vi "Process.vi"(8 "error in":errorcluster, 11 "Chart[Template]":refnum<class "Chart[Template].lvclass">) -> (0 "error out":errorcluster, 3 "Graph[Template] out":refnum<class "Chart[Template].lvclass">)   [LabVIEW 2013, in "Chart[Template].lvclass"]
doc: "---------------------------------------------------------------\nJKI State Machine Objects™\nhttp://jki.net/state-machine-objects/\nCopyright (C) 2005-2015, JKI <info@jki.net>\nALL RIGHTS RESERVEDJKI State Machine Objects (SMO) 1.0.0.5\nJKI - JKI\nCopyright (c) 2016, JKI"
uses:
  Chart[Template].lvclass
  <vilib>/JKI/JKI SMO/SMO/Typedefs/Parent Call--Enum.ctl
  <vilib>/JKI/JKI SMO/SMO.UI/SMO.UI.lvclass
  Chart[Template].lvclass/Chart[Template].ctl
  <vilib>/JKI/JKI SMO/SMO/SMO.lvclass
panel:
  in  "------------- Registered Events -------------":bool
  in  "------------- Public API -------------":bool
  out "Waveform Chart":dbl(graph)
  # "For instructions on how to use the JKI State Machine Objects, examples and video tutorials, visit:\nhttp://jki.net/state-machine-objects/\n\nJKI State Machine Objects™\nhttp://jki.net/state-machine-objects/\nCopyright (C) 2005-2015, JKI <info@jki.net>\nALL RIGHTS RESERVED"
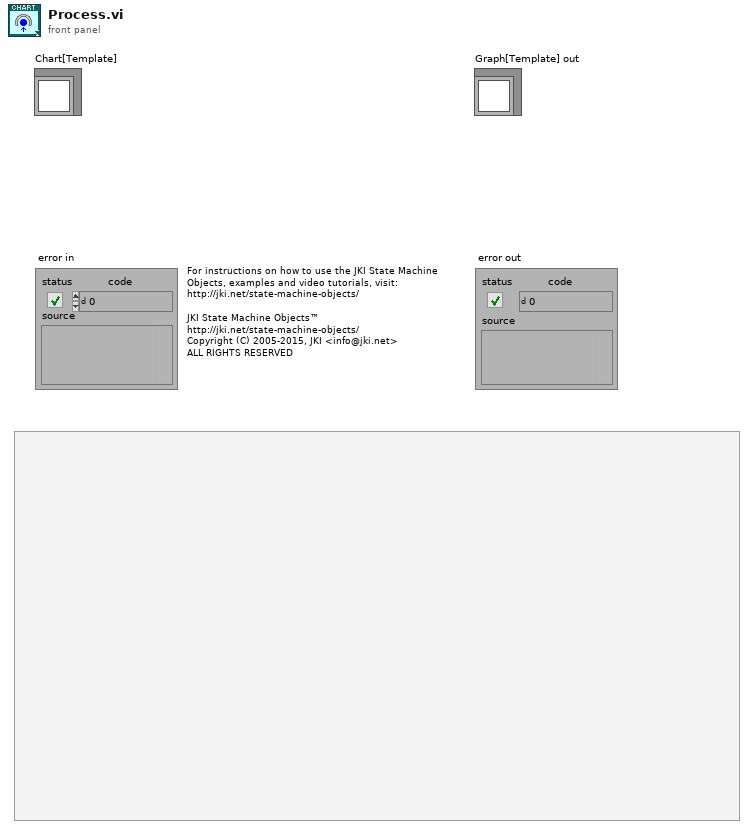
[diagram p1: front panel]
types:
  T1 = typedef "SMO.lvclass/Parent Call--Enum.ctl" = enum16{"Allows parent to run", "Does not request parent to run"}
  T2 = enum32{"invalid app kind", "Development System", "Run Time System", "Student Edition", "Embedded LabVIEW", "Evaluation", "Custom"}
  T3 = enum32{"Invalid", "Standard", "Closed", "Hidden", "Minimized", "Maximized"}
  T4 = cluster{"Core":cluster{"Current VI Reference":refnum<vi>, "Close Panel on Exit?":bool, "error":errorcluster}, "Self Reference":refnum<class "Chart[Template].lvclass">, "bool":bool}
  T5 = cluster{"Current VI Reference":refnum<vi>, "Close Panel on Exit?":bool, "error":errorcluster}
  T6 = typedef "SMO.lvclass/Protected Events.ctl" = cluster{"StopProcesses":refnum<user-event>, "AbortProcesses":refnum<user-event>, "Config Changed":refnum<user-event>}
  T7 = typedef "Chart[Template].lvclass/ProtectedEvents--Cluster.ctl" = cluster{"Clear Chart":refnum<user-event>}
  T8 = typedef "Chart[Template].lvclass/Dependencies--Cluster.ctl" = cluster{"SMO":refnum<class "SMO.lvclass">, "New Value":refnum<user-event>}
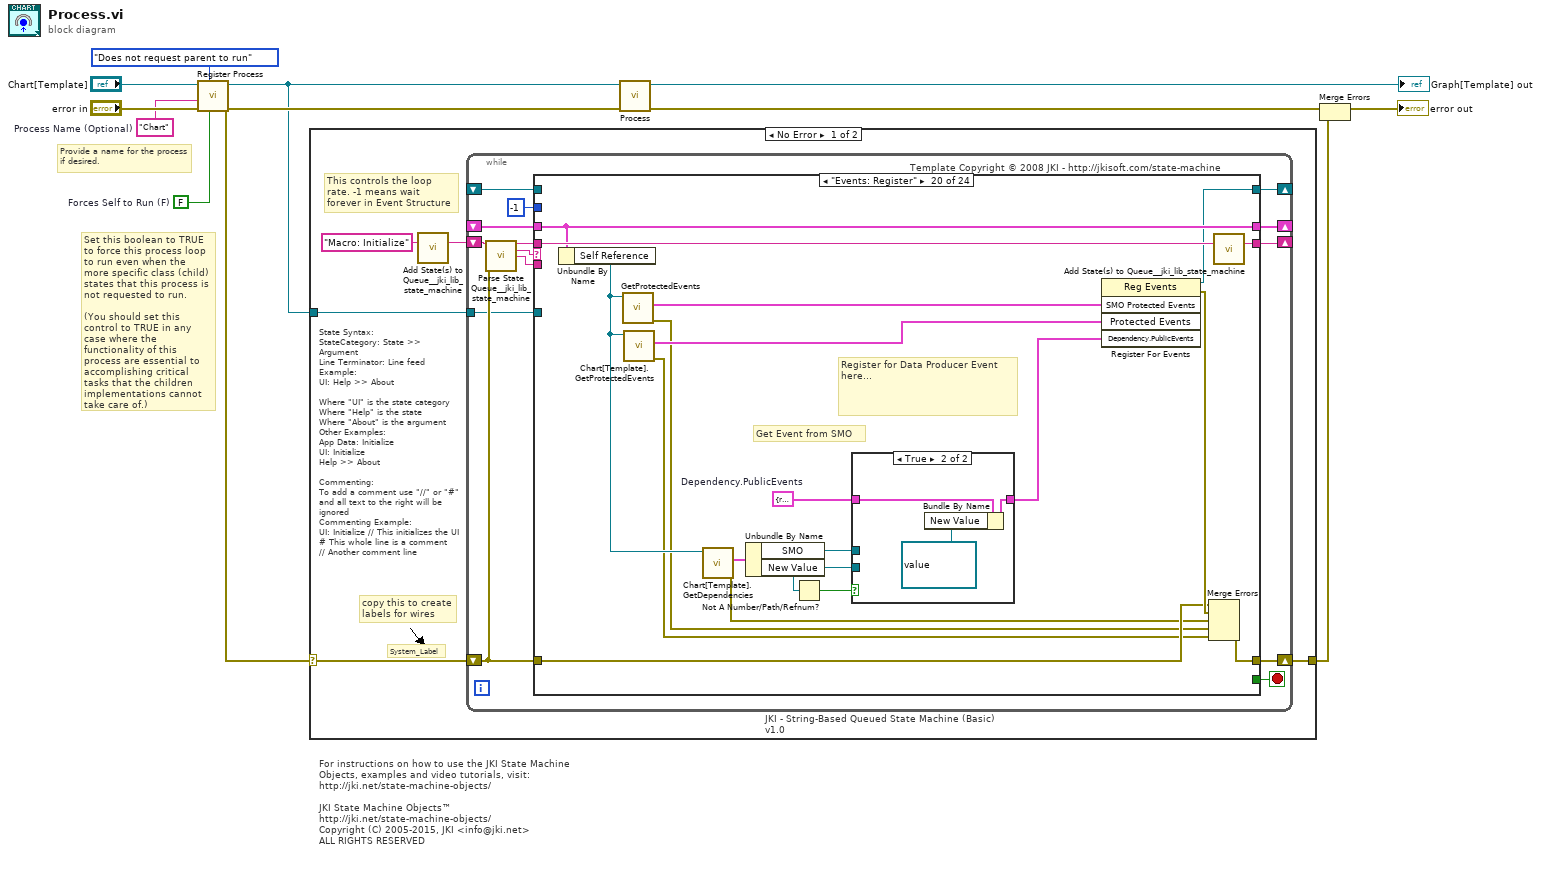
[diagram p0: block diagram]
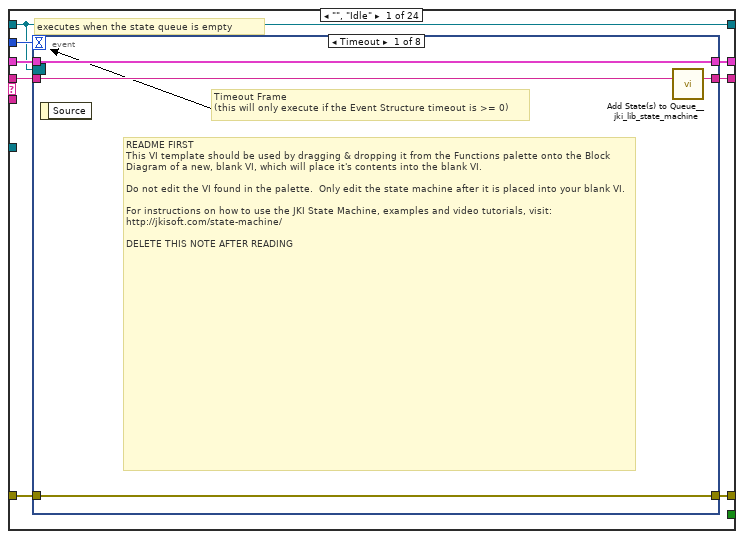
[diagram p2: hidden frame]
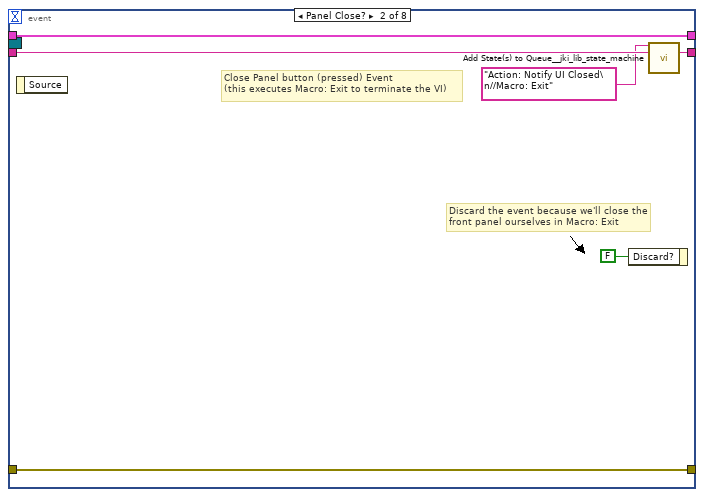
[diagram p3: hidden frame]
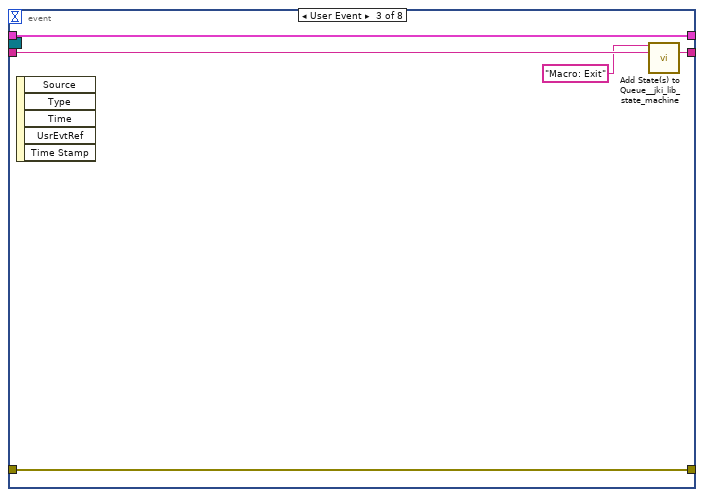
[diagram p4: hidden frame]
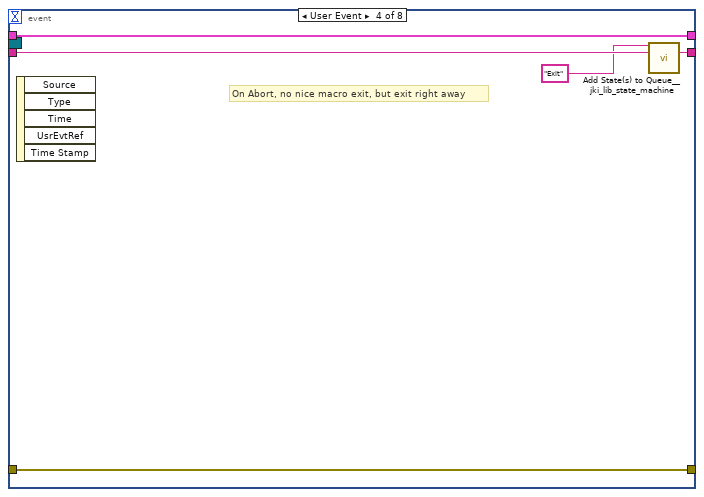
[diagram p5: hidden frame]
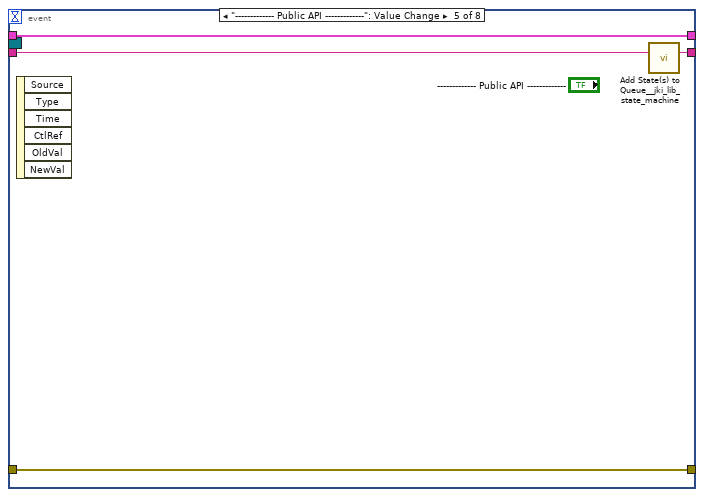
[diagram p6: hidden frame]
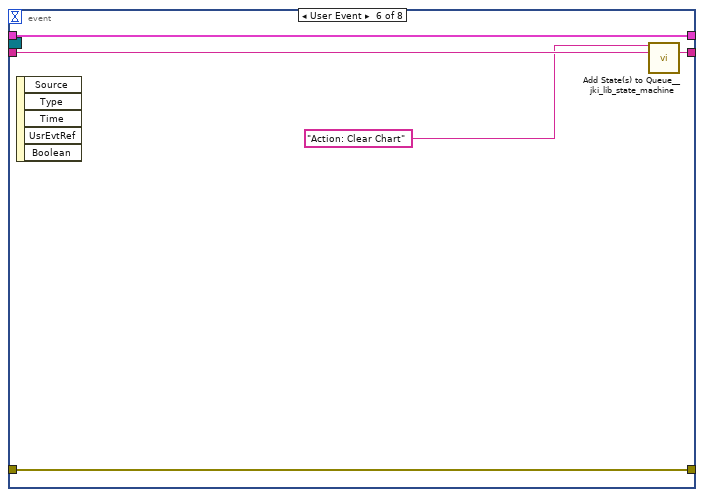
[diagram p7: hidden frame]
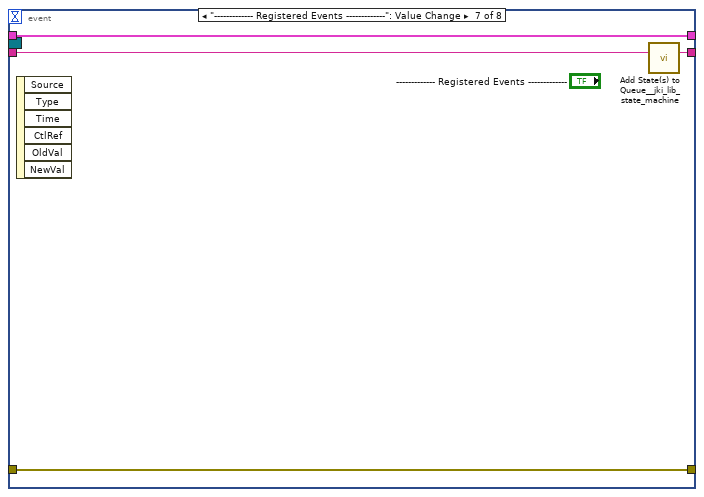
[diagram p8: hidden frame]
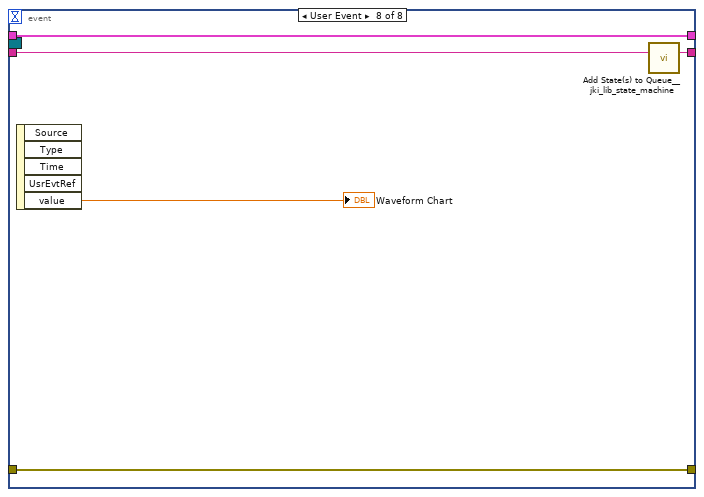
[diagram p9: hidden frame]
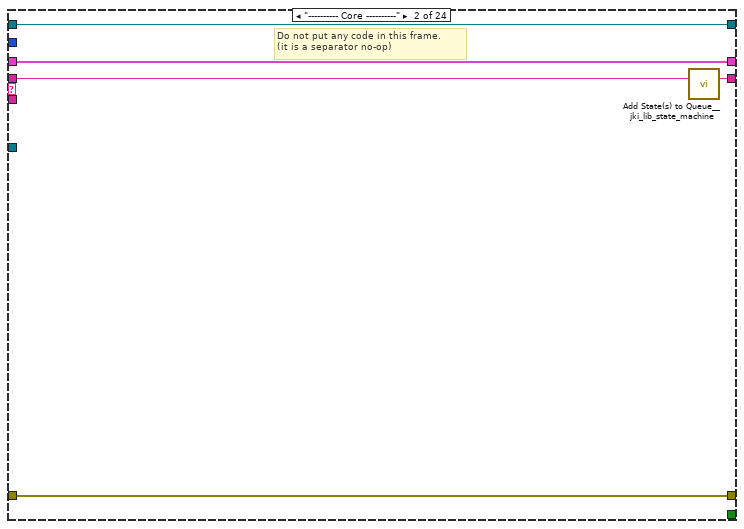
[diagram p10: hidden frame]
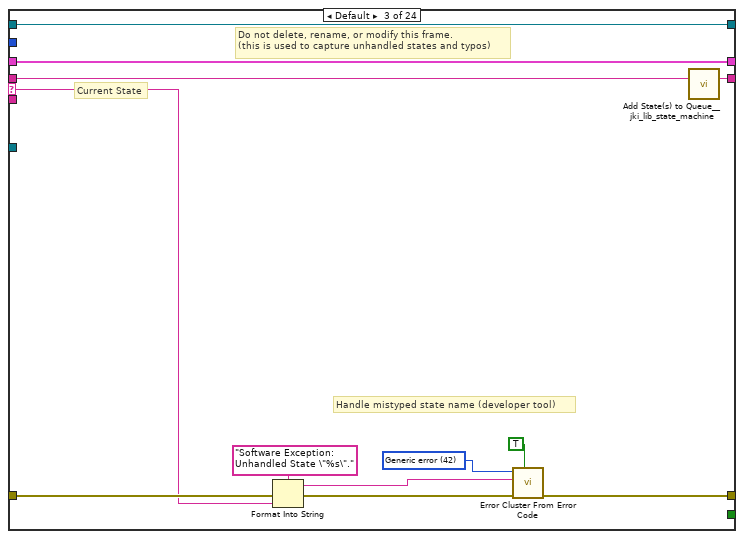
[diagram p11: hidden frame]
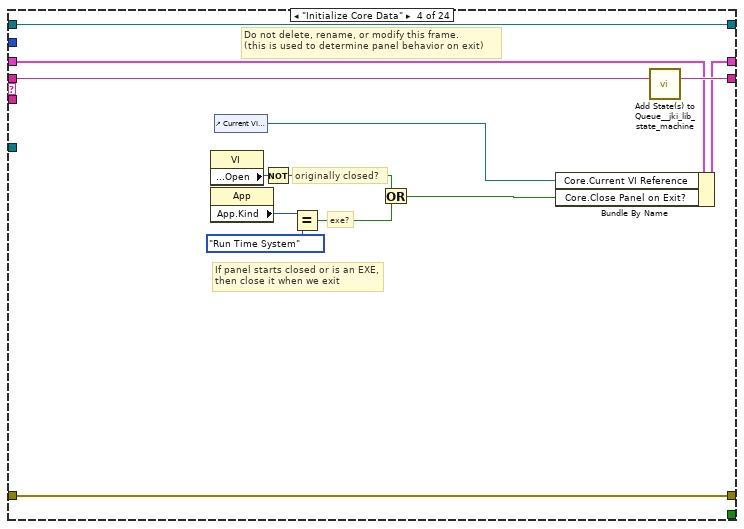
[diagram p12: hidden frame]
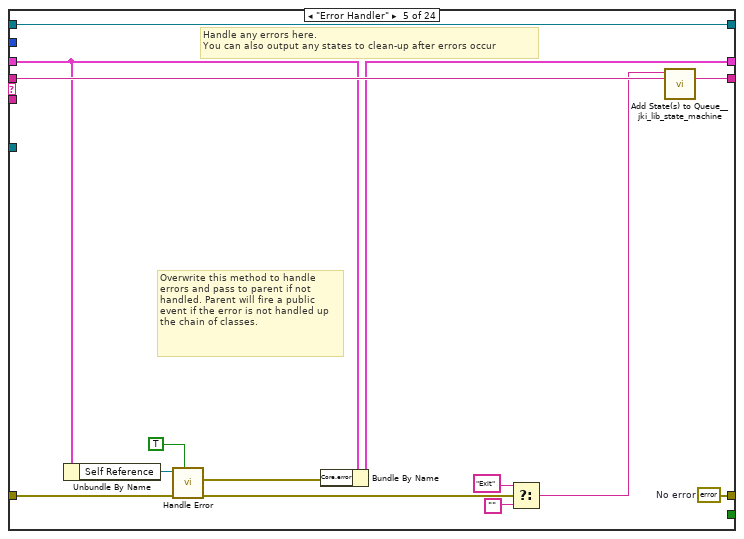
[diagram p13: hidden frame]
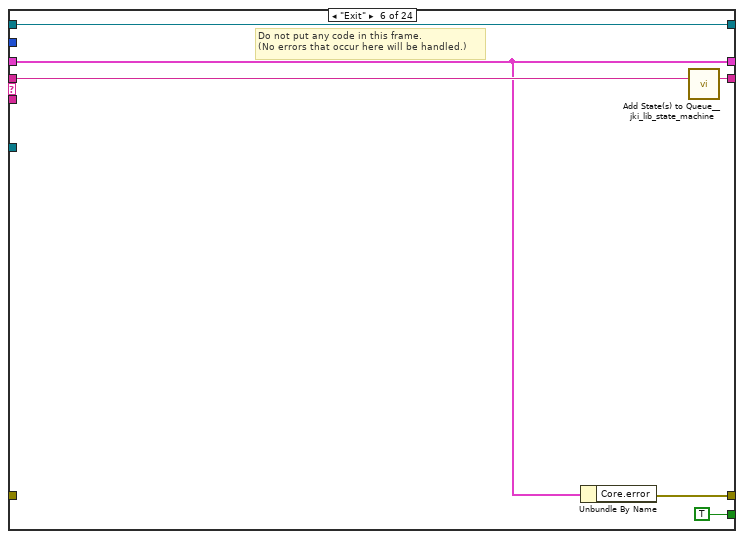
[diagram p14: hidden frame]
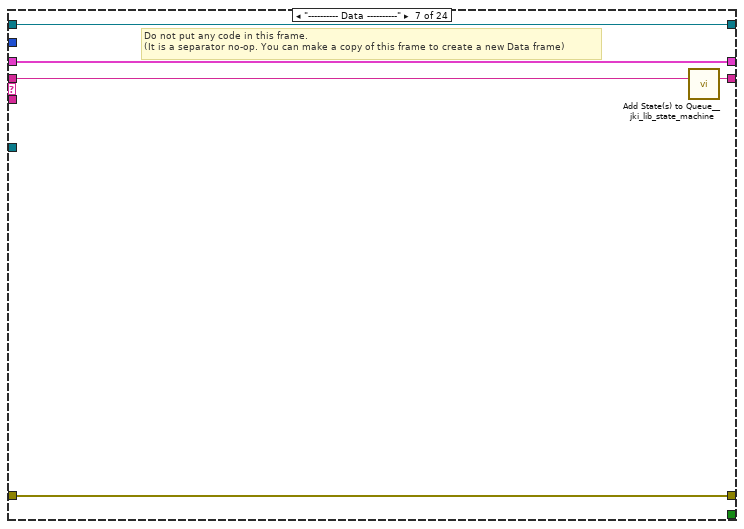
[diagram p15: hidden frame]
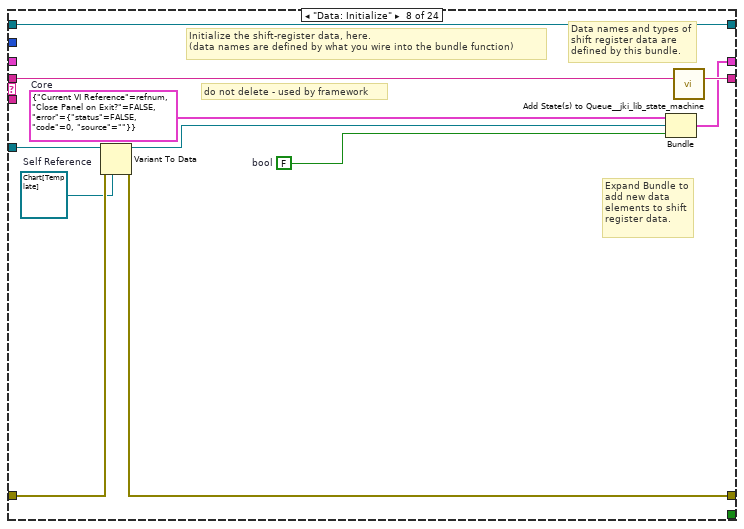
[diagram p16: hidden frame]
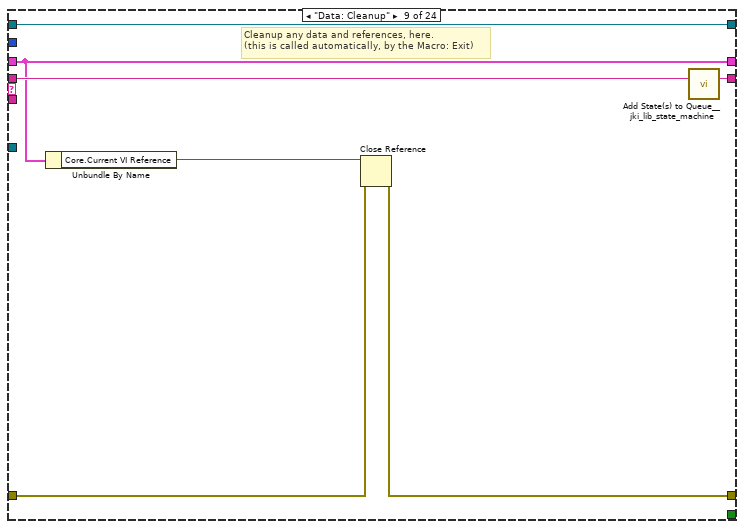
[diagram p17: hidden frame]
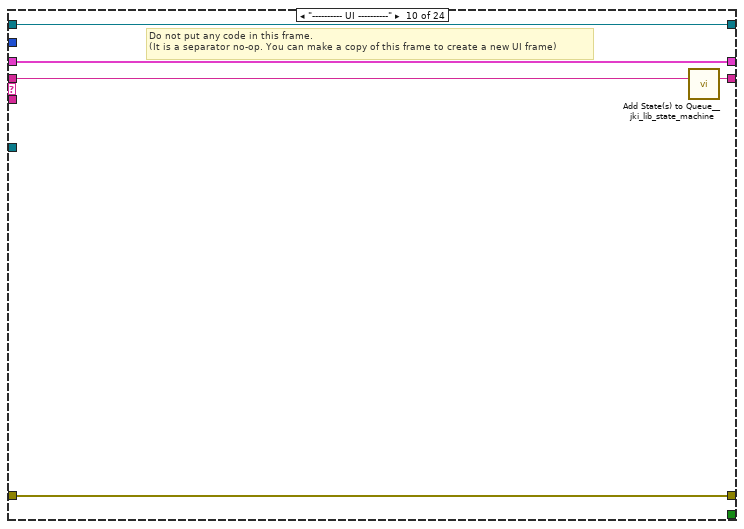
[diagram p18: hidden frame]
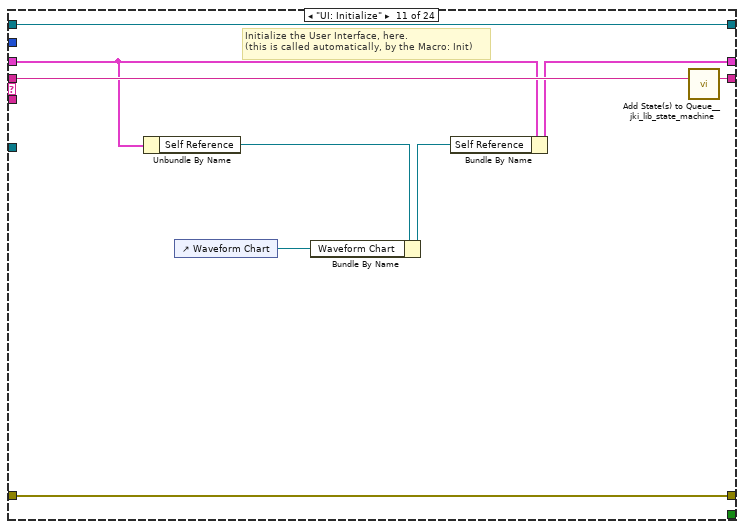
[diagram p19: hidden frame]
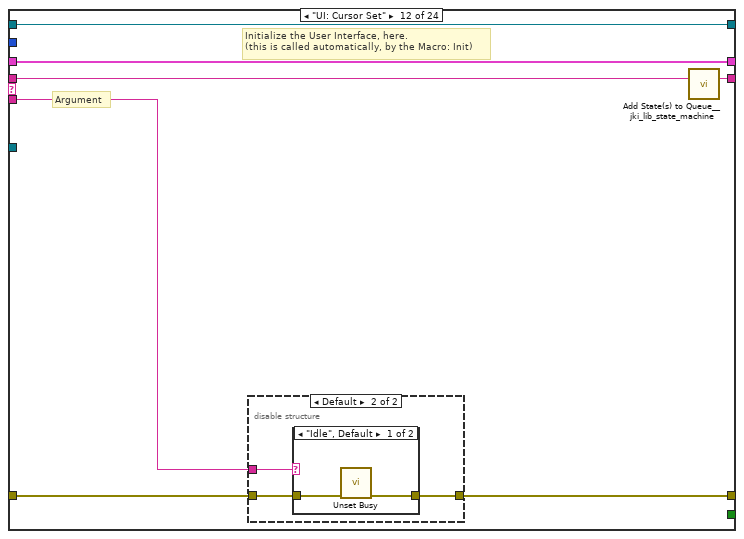
[diagram p20: hidden frame]
diagram:
  w2 = FALSE  # Forces Self to Run (F)
  w1 = "Chart"  # Process Name (Optional)
  # "Provide a name for the process\nif desired."
  # "Set this boolean to TRUE to force this process loop to run even when the more specific class (child) states that this process is not requested to run.\n\n(You should set this control to TRUE in any case where the functionality of this process are essential to accomplishing critical tasks that the children implementations cannot take care of.)"
  # "For instructions on how to use the JKI State Machine Objects, examples and video tutorials, visit:\nhttp://jki.net/state-machine-objects/\n\nJKI State Machine Objects™\nhttp://jki.net/state-machine-objects/\nCopyright (C) 2005-2015, JKI <info@jki.net>\nALL RIGHTS RESERVED"
  n1 = call <vilib>:"Register Process.vi"("Forces Self to Run (F)"=w2, "Parent Call"=Parent_Call--Enum."Does not request parent to run", "error in (no error)"="error in", "Process Name (optional)"=w1, "SMO"="Chart[Template]") -> ("error out"=w8:errorcluster, "SMO out"=w7:refnum<class "Chart[Template].lvclass">)  [unwired: 5 in]
  n2 = case shown="No Error" w8 {
    selector: w8 -> [w13 w313]
    tunnel: w7 -> [w14 _]
    tunnel: [w12 w313] -> w4
    frame No Error {
      # "State Syntax:\nStateCategory: State >> Argument\nLine Terminator: Line feed\nExample:\nUI: Help >> About\n\nWhere \"UI\" is the state category\nWhere \"Help\" is the state\nWhere \"About\" is the argument\nOther Examples:\nApp Data: Initialize\nUI: Initialize\nHelp >> About\n\nCommenting:\nTo add a comment use \"//\" or \"#\" and all text to the right will be ignored\nCommenting Example:\nUI: Initialize // This initializes the UI\n# This whole line is a comment\n// Another comment line"
      # "copy this to create labels for wires"
      # "This controls the loop rate. -1 means wait forever in Event Structure"
      # "System_Label"
      n3 = call <vilib>:"Add State(s) to Queue__jki_lib_state_machine.vi"("State(s) in (\"\")"="Macro: Initialize") -> ("States Out"=w16:string)  [unwired: 14 in]
      n4 = while "JKI - String-Based Queued State Machine (Basic) v1.0" {
        shift-right: [w23] -> _
        shift-left: _ -> [w22]
        shift-right: [w26] -> w12
        shift-left: w13 -> [w20]
        shift-right: [w25] -> _
        shift-left: w16 -> [w27]
        tunnel: w14 -> [w19]
        shift-right: [w18] -> _
        shift-left: _ -> [w17]
        stop <- w24 stop-if-true
        # "Template Copyright © 2008 JKI - http://jkisoft.com/state-machine"
        n5 = call <vilib>:"Parse State Queue__jki_lib_state_machine.vi"("State Queue"=w27, "Error In (no error)"=w20) -> ("Remaining States"=w29:string, "Current State"=w30:string, "Arguments"=w28:string)  [unwired: 11 in]
        n6 = case shown="\"Events: Register\"" w30 {
          selector: w30 -> [_ _ w83 _ _ _ _ _ _ _ _ _ _ _ _ _ _ _ _ _ _ _ _ _]
          tunnel: w29 -> [w38 w81 w87 w106 w120 w126 w131 w142 w149 w154 w163 w170 w186 w218 w227 w241 w246 w257 w262 w281 w293 w298 w305 w312]
          tunnel: w28 -> [_ _ _ _ _ _ _ _ _ _ _ w164 w180 _ _ _ _ _ _ _ _ _ _ _]
          tunnel: w22 -> [w36 w78 w85 w97 w109 w122 w128 _ w144 w151 w159 w168 w182 w215 w223 w232 w243 w254 w259 w279 w291 w296 w302 w308]
          tunnel: [w35 w79 w89 w103 w111 w121 w129 w137 w145 w152 w161 w165 w183 w216 w225 w239 w244 w248 w260 w276 w289 w294 w300 w306] -> w26
          tunnel: w20 -> [w34 w79 w88 w103 w116 _ w129 w138 w146 w152 w161 w166 w184 w216 w225 w239 w244 w249 w260 w271 w289 w294 w301 w307]
          tunnel: [w37 w80 w86 w105 w119 w125 w130 w141 w148 w153 w162 w169 w185 w217 w226 w240 w245 w256 w261 w280 w292 w297 w304 w311] -> w25
          tunnel: [_ _ _ _ _ TRUE _ _ _ _ _ _ _ _ _ _ _ _ _ _ _ _ _ _] -> w24
          tunnel: [w33 w78 w85 w104 w108 w122 w128 w140 w144 w151 w158 w168 w182 w215 w223 w232 w243 w254 w259 w279 w291 w296 w302 w308] -> w23
          tunnel: -1 ("Timeout") -> [w32 _ _ _ _ _ _ _ _ _ _ _ _ _ _ _ _ _ _ _ _ _ _ _]
          tunnel: w19 -> [_ _ _ _ _ _ _ w135 _ _ _ _ _ _ _ _ _ _ _ _ _ _ _ _]
          tunnel: [w31 w77 w82 w94 w118 w123 w127 w133 w143 w150 w160 w167 w179 w214 w224 w233 w242 w255 w258 w278 w290 w295 w303 w310] -> w18
          tunnel: w17 -> [w31 w77 w82 w94 w118 w123 w127 w133 w143 w150 w160 w167 w179 w214 w224 w233 w242 w255 w258 _ w290 w295 w303 w310]
          frame "", "Idle" {
            # "executes when the state queue is empty"
            n7 = event shown="[0] Timeout" {
              selector: w31 -> [_ _ _ _ _ _ _ _]
              dyn-events: _ -> [_ _ _ _ _ _ _ _]
              timeout: w32 -> [_ _ _ _ _ _ _ _]
              tunnel: w38 -> [w42 w48 w53 w58 w62 w67 w71 w76]
              tunnel: [w41 w47 w52 w57 w61 w66 w70 w75] -> w37
              tunnel: w36 -> [w39 w44 w50 w55 w59 w64 w68 w73]
              tunnel: [w40 w43 w51 w56 w60 w65 w69 w74] -> w35
              tunnel: w34 -> [w40 w43 w51 w56 w60 w65 w69 w74]
              tunnel: [w39 w44 w50 w55 w59 w64 w68 w73] -> w33
              event Timeout {
                # "README FIRST\nThis VI template should be used by dragging & dropping it from the Functions palette onto the Block Diagram of a new, blank VI, which will place it's contents into the blank VI.\n\nDo not edit the VI found in the palette.  Only edit the state machine after it is placed into your blank VI.\n\nFor instructions on how to use the JKI State Machine, examples and video tutorials, visit:\nhttp://jkisoft.com/state-machine/\n\nDELETE THIS NOTE AFTER READING"
                # "Timeout Frame\n(this will only execute if the Event Structure timeout is >= 0)"
                n8 = event-data() -> ()  [unwired: 1 in, 1 out]
                n9 = call <vilib>:"Add State(s) to Queue__jki_lib_state_machine.vi"("State(s) in (\"\")"=w42) -> ("States Out"=w41:string)  [unwired: 14 in]
              }
              event Panel Close? {
                # "Discard the event because we'll close the front panel ourselves in Macro: Exit"
                # "Close Panel button (pressed) Event\n(this executes Macro: Exit to terminate the VI)"
                n10 = event-data() -> ()  [unwired: 1 in, 1 out]
                n11 = event-data("Discard?"=FALSE) -> ()  [unwired: 1 in, 1 out]
                n12 = call <vilib>:"Add State(s) to Queue__jki_lib_state_machine.vi"("State(s) in Front (\"\")"="Action: Notify UI Closed\n//Macro: Exit", "State(s) in (\"\")"=w48) -> ("States Out"=w47:string)  [unwired: 13 in]
              }
              event User Event {
                n13 = event-data() -> ()  [unwired: 1 in, 5 out]
                n14 = call <vilib>:"Add State(s) to Queue__jki_lib_state_machine.vi"("State(s) in Front (\"\")"="Macro: Exit", "State(s) in (\"\")"=w53) -> ("States Out"=w52:string)  [unwired: 13 in]
              }
              event User Event {
                # "On Abort, no nice macro exit, but exit right away"
                n15 = event-data() -> ()  [unwired: 1 in, 5 out]
                n16 = call <vilib>:"Add State(s) to Queue__jki_lib_state_machine.vi"("State(s) in Front (\"\")"="Exit", "State(s) in (\"\")"=w58) -> ("States Out"=w57:string)  [unwired: 13 in]
              }
              event "------------- Public API -------------": Value Change {
                n17 = event-data() -> ()  [unwired: 1 in, 6 out]
                n18 = call <vilib>:"Add State(s) to Queue__jki_lib_state_machine.vi"("State(s) in (\"\")"=w62) -> ("States Out"=w61:string)  [unwired: 14 in]
              }
              event User Event {
                n19 = event-data() -> ()  [unwired: 1 in, 5 out]
                n20 = call <vilib>:"Add State(s) to Queue__jki_lib_state_machine.vi"("State(s) in Front (\"\")"="Action: Clear Chart", "State(s) in (\"\")"=w67) -> ("States Out"=w66:string)  [unwired: 13 in]
              }
              event "------------- Registered Events -------------": Value Change {
                n21 = event-data() -> ()  [unwired: 1 in, 6 out]
                n22 = call <vilib>:"Add State(s) to Queue__jki_lib_state_machine.vi"("State(s) in (\"\")"=w71) -> ("States Out"=w70:string)  [unwired: 14 in]
              }
              event User Event {
                n23 = event-data() -> ("value"=→"Waveform Chart":dbl)  [unwired: 1 in, 4 out]
                n24 = call <vilib>:"Add State(s) to Queue__jki_lib_state_machine.vi"("State(s) in (\"\")"=w76) -> ("States Out"=w75:string)  [unwired: 14 in]
              }
            }
          }
          frame "---------- Core ----------" {
            # "Do not put any code in this frame.\n(it is a separator no-op)"
            n25 = call <vilib>:"Add State(s) to Queue__jki_lib_state_machine.vi"("State(s) in (\"\")"=w81) -> ("States Out"=w80:string)  [unwired: 14 in]
          }
          frame Default {
            w92 = 42 items=["No error", "Argument error", "Memory is full", "Out of zone", "End of file", "File already open", "Generic file I/O error", "File not found", "File permission error", "Disk is full", "Duplicate path", "Too many files open", "System feature not enabled", "Resource file not found", "Cannot add resource", "Resource not found", "Image not found", "Image memory error", "Pen does not exist", "Config type invalid", "Config token not found", "Config parse error", "Config memory error", "Bad external code format", "Bad external code offset", "External code not present", "Null window", "Destroy window error", "Null menu", "Print aborted", "Bad print record", "Print driver error", "Windows error during printing", "Memory error during printing", "Print dialog error", "Generic print error", "Invalid device refnum", "Device not found", "Device parameter error", "Device unit error", "Cannot open device", "Device call aborted", "Generic error", "Cancelled by user", "Object ID too low", "Object ID too high", "Object not in heap", "Unknown heap", "Unknown object (invalid DefProc)", "Unknown object (DefProc not in table)", "Message out of range", "Invalid (null) method", "Unknown message", "Manager call not supported", "Bad address", "Network operation in progress", "Network operation timed out", "Connection is busy", "Network attribute not supported", "Network error", "Address in use", "System out of memory", "Connection aborted", "Connection refused", "Not connected", "Already connected", "Connection closed", "Initialization error (interapplication manager)", "Bad occurrence", "Wait on unbound occurrence handler", "Occurrence queue overflow", "Datalog type conflict", "Unused", "Unrecognized type (interapplication manager)", "Memory corrupt", "Failed to make temporary DLL", "Old CIN version", "Drag socket not found", "Failed to load drop-object", "Failed to register OLE object", "Failed to release OLE object", "Format specifier type mismatch", "Unknown format specifier", "Too few format specifiers", "Too many format specifiers", "Scan failed", "Newer CIN version", "Error converting to variant", "Runtime menu error", "Password tampered", "Variant attribute not found", "Incompatible variant data type", "Event data is not available", "Event Store is not present", "Occurrence is not found", "Event Queue is not created", "Event info is not available", "Refnum passed is NULL", "Error retrieving Class GUID", "Error retrieving CoClass GUID", "Error retrieving TypeLib GUID.", "Bad built application magic bytes.", "Specific driver is different from the specific driver associated with the Logical Name.", "There is no session opened to the class driver.", "Max Error", "MAX - Error with config objects", "MAX - Error loading configuration", "MAX - Group not supported"]
            # "Current State"
            # "Do not delete, rename, or modify this frame.\n(this is used to capture unhandled states and typos)"
            # "Handle mistyped state name (developer tool)"
            n26 = Format Into String(format string="Software Exception: Unhandled State \"%s\"." ("message"), error in=w88, w83) -> (resulting string=w91:string, error out=w90:errorcluster)  [unwired: 1 in]
            n27 = call <vilib>:"Error Cluster From Error Code.vi"("show call chain? (False)"=TRUE, "error in (no error)"=w90, "error message (\"\")"=w91, "error code (0)"=w92) -> ("error out"=w89:errorcluster)  [unwired: 5 in]
            n28 = call <vilib>:"Add State(s) to Queue__jki_lib_state_machine.vi"("State(s) in (\"\")"=w87) -> ("States Out"=w86:string)  [unwired: 14 in]
          }
          frame "Initialize Core Data" {
            # "Do not delete, rename, or modify this frame.\n(this is used to determine panel behavior on exit)"
            # "originally closed?"
            # "exe?"
            # "If panel starts closed or is an EXE, then close it when we exit"
            n29 = property class="VI"() -> ("Front Panel.Open"=w102:bool)  [unwired: 2 in, 2 out]
            n30 = property class="App"() -> ("App.Kind"=w101:T2)  [unwired: 2 in, 2 out]
            n31 = control-ref of="Current VI Reference"() -> (w95:refnum<vi>)
            n32 = Not(x=w102) -> (.not. x?=w99:bool)
            n33 = Equal?(x=w101, y=T2."Run Time System" ("Application:Kind")) -> (x = y?=w98:bool)
            n34 = Or(x=w99, y=w98) -> (x .or. y?=w96:bool)
            n35 = Bundle By Name(cluster=w97, "Core.Current VI Reference"=w95, "Core.Close Panel on Exit?"=w96) -> (w104:T4)
            n36 = call <vilib>:"Add State(s) to Queue__jki_lib_state_machine.vi"("State(s) in (\"\")"=w106) -> ("States Out"=w105:string)  [unwired: 14 in]
          }
          frame "Error Handler" {
            w111 = errorcluster {"status"=FALSE, "code"=0, "source"=""}  # No error
            # "Overwrite this method to handle errors and pass to parent if not handled. Parent will fire a public event if the error is not handled up the chain of classes."
            # "Handle any errors here.\nYou can also output any states to clean-up after errors occur"
            n37 = Unbundle By Name(w109) -> ("Self Reference"=w117:refnum<class "Chart[Template].lvclass">)
            n38 = call-dynamic "Handle Error.vi"("Stop on Unhandled Error (T)"=TRUE, "error in"=w116, "SMO"=w117) -> ("handling error"=w112:errorcluster, "Unhandled error"=w110:errorcluster)  [unwired: 6 in, 1 out]
            n39 = Bundle By Name(cluster=w109, "Core.error"=w110) -> (w108:T4)
            n40 = Select(t="Exit", s=w112, f="") -> (s? t:f=w113:string)
            n41 = call <vilib>:"Add State(s) to Queue__jki_lib_state_machine.vi"("State(s) in Front (\"\")"=w113, "State(s) in (\"\")"=w120) -> ("States Out"=w119:string)  [unwired: 13 in]
          }
          frame "Exit" {
            # "Do not put any code in this frame.\n(No errors that occur here will be handled.)"
            n42 = Unbundle By Name(w122) -> ("Core.error"=w121:errorcluster)
            n43 = call <vilib>:"Add State(s) to Queue__jki_lib_state_machine.vi"("State(s) in (\"\")"=w126) -> ("States Out"=w125:string)  [unwired: 14 in]
          }
          frame "---------- Data ----------" {
            # "Do not put any code in this frame.\n(It is a separator no-op. You can make a copy of this frame to create a new Data frame)"
            n44 = call <vilib>:"Add State(s) to Queue__jki_lib_state_machine.vi"("State(s) in (\"\")"=w131) -> ("States Out"=w130:string)  [unwired: 14 in]
          }
          frame "Data: Initialize" {
            w132 = T5 {"Current VI Reference"=refnum, "Close Panel on Exit?"=FALSE, "error"={"status"=FALSE, "code"=0, "source"=""}}  # Core
            w136 = refnum<class "Chart[Template].lvclass"> refnum  # Self Reference
            w139 = FALSE  # bool
            # "do not delete - used by framework"
            # "Expand Bundle to add new data elements to shift register data."
            # "Data names and types of shift register data are defined by this bundle."
            # "Initialize the shift-register data, here.\n(data names are defined by what you wire into the bundle function)"
            n45 = Variant To Data(error in=w138, type=w136, Variant=w135) -> (data=w134:refnum<class "Chart[Template].lvclass">, error out=w137:errorcluster)
            n46 = Bundle("Core"=w132, "Self Reference"=w134, "bool"=w139) -> (w140:T4)  [unwired: 1 in]
            n47 = call <vilib>:"Add State(s) to Queue__jki_lib_state_machine.vi"("State(s) in (\"\")"=w142) -> ("States Out"=w141:string)  [unwired: 14 in]
          }
          frame "Data: Cleanup" {
            # "Cleanup any data and references, here.\n(this is called automatically, by the Macro: Exit)"
            n48 = Unbundle By Name(w144) -> ("Core.Current VI Reference"=w147:refnum<vi>)
            n49 = Close Reference(reference=w147, error in (no error)=w146) -> (error out=w145:errorcluster)
            n50 = call <vilib>:"Add State(s) to Queue__jki_lib_state_machine.vi"("State(s) in (\"\")"=w149) -> ("States Out"=w148:string)  [unwired: 14 in]
          }
          frame "---------- UI ----------" {
            # "Do not put any code in this frame.\n(It is a separator no-op. You can make a copy of this frame to create a new UI frame)"
            n51 = call <vilib>:"Add State(s) to Queue__jki_lib_state_machine.vi"("State(s) in (\"\")"=w154) -> ("States Out"=w153:string)  [unwired: 14 in]
          }
          frame "UI: Initialize" {
            # "Initialize the User Interface, here.\n(this is called automatically, by the Macro: Init)"
            n52 = Unbundle By Name(w159) -> ("Self Reference"=w157:refnum<class "Chart[Template].lvclass">)
            n53 = control-ref of="Waveform Chart"() -> (w156:refnum<vi>)
            n54 = Bundle By Name(cluster=w157, "Waveform Chart"=w156) -> (w155:refnum<class "Chart[Template].lvclass">)
            n55 = Bundle By Name(cluster=w159, "Self Reference"=w155) -> (w158:T4)
            n56 = call <vilib>:"Add State(s) to Queue__jki_lib_state_machine.vi"("State(s) in (\"\")"=w163) -> ("States Out"=w162:string)  [unwired: 14 in]
          }
          frame "UI: Cursor Set" {
            # "Argument"
            # "Initialize the User Interface, here.\n(this is called automatically, by the Macro: Init)"
            n57 = disable-structure shown="Default" {
              disable-tunnel: w166 -> [w171 w174]
              disable-tunnel: [w171 w173] -> w165
              disable-tunnel: w164 -> [_ w172]
              frame condition #0 {
              }
              frame condition #1 (active) {
                n58 = case shown="\"Idle\", Default" w172 {
                  tunnel: w174 -> [w176 w178]
                  tunnel: [w175 w177] -> w173
                  frame "Idle", Default {
                    n59 = call <vilib>:"Unset Busy.vi"("error in (no error)"=w176) -> ("error out"=w175:errorcluster)  [unwired: 10 in]
                  }
                  frame "Busy" {
                    n60 = call <vilib>:"Set Busy.vi"("error in (no error)"=w178) -> ("error out"=w177:errorcluster)  [unwired: 9 in, 1 out]
                  }
                }
              }
            }
            n61 = call <vilib>:"Add State(s) to Queue__jki_lib_state_machine.vi"("State(s) in (\"\")"=w170) -> ("States Out"=w169:string)  [unwired: 14 in]
          }
          frame "UI: Front Panel State" {
            # "Argument"
            # "Set Front Panel Open or Closed\n(Usage: \"UI: Front Panel State >> Open|Close\")"
            n62 = Unbundle By Name(w182) -> ("Core.Current VI Reference"=w181:refnum<vi>)
            n63 = disable-structure shown="Default" {
              disable-tunnel: w184 -> [w190 w213]
              disable-tunnel: [w189 w213] -> w183
              disable-tunnel: w181 -> [w188 _]
              disable-tunnel: w180 -> [w187 _]
              frame condition #0 (active) {
                n64 = case shown="\"Close\"" w187 {
                  tunnel: w190 -> [w194 w207]
                  tunnel: [w196 w208] -> w189
                  tunnel: w188 -> [w195 w205]
                  frame "Open", Default {
                    n65 = property class="VI"(reference=w195, error in=w194) -> (reference out=w192:refnum<vi>, error out=w193:errorcluster, "FP.State"=w191:T3)
                    n66 = case shown="\"Closed\"" w191 {
                      tunnel: [w199 w202] -> w196
                      tunnel: w193 -> [w198 w202]
                      tunnel: w192 -> [w197 _]
                      frame "Closed" {
                        n67 = invoke class="VI" method="FP.Open"(reference=w197, error in=w198, "Activate"=TRUE, "State"=T3."Standard") -> (error out=w199:errorcluster)  [unwired: 1 in, 4 out]
                      }
                      frame Default {
                      }
                    }
                  }
                  frame "Close" {
                    n68 = property class="VI"(reference=w205, error in=w207) -> (reference out=w204:refnum<vi>, error out=w206:errorcluster, "FP.State"=w203:T3)
                    n69 = case shown="Default" w203 {
                      tunnel: [w209 w212] -> w208
                      tunnel: w206 -> [w209 w211]
                      tunnel: w204 -> [_ w210]
                      frame "Invalid", "Closed" {
                      }
                      frame Default {
                        n70 = invoke class="VI" method="FP.Close"(reference=w210, error in=w211) -> (error out=w212:errorcluster)  [unwired: 1 in, 2 out]
                      }
                    }
                  }
                }
              }
              frame condition #1 {
              }
            }
            n71 = call <vilib>:"Add State(s) to Queue__jki_lib_state_machine.vi"("State(s) in (\"\")"=w186) -> ("States Out"=w185:string)  [unwired: 14 in]
          }
          frame "---------- Macro ----------" {
            # "Do not put any code in this frame.\n(It is a separator no-op. You can make a copy of this frame to create a new Macro frame)"
            n72 = call <vilib>:"Add State(s) to Queue__jki_lib_state_machine.vi"("State(s) in (\"\")"=w218) -> ("States Out"=w217:string)  [unwired: 14 in]
          }
          frame "Macro: Initialize" {
            w221 = "UI: Initialize\n//UI: Front Panel State >> Open"  # UI: Initialize //UI: Front Panel State >> Open
            # "Initialization Macro\n(This is called once, when the VI starts)"
            n73 = call <vilib>:"Add State(s) to Queue__jki_lib_state_machine.vi"("State(s) in Front (\"\")"="Data: Initialize\nInitialize Core Data\nEvents: Register", "State(s) in (\"\")"="Process: Sync", "State(s) at Back (\"\")"=w221) -> ("States Out"=w220:string)  [unwired: 12 in]
            n74 = call <vilib>:"Add State(s) to Queue__jki_lib_state_machine.vi"("State(s) in Front (\"\")"=w220, "State(s) in (\"\")"=w227) -> ("States Out"=w226:string)  [unwired: 13 in]
          }
          frame "Macro: Exit" {
            # "Exit Macro\n(This is called once, when the VI exits)"
            n75 = Unbundle By Name(w232) -> ("Core.Close Panel on Exit?"=w238:bool)
            n76 = Select(t="//UI: Front Panel State >> Close", s=w238, f="") -> (s? t:f=w235:string)
            n77 = call <vilib>:"Add State(s) to Queue__jki_lib_state_machine.vi"("State(s) in Front (\"\")"="Data: Cleanup\nEvents: Unregister", "State(s) in (\"\")"="Process: Sync", "State(s) at Back (\"\")"="Exit") -> ("States Out"=w229:string)  [unwired: 12 in]
            n78 = call <vilib>:"Add State(s) to Queue__jki_lib_state_machine.vi"("State(s) in (\"\")"=w235, "State(s) at Back (\"\")"=w229) -> ("States Out"=w234:string)  [unwired: 13 in]
            n79 = call <vilib>:"Add State(s) to Queue__jki_lib_state_machine.vi"("State(s) in Front (\"\")"=w234, "State(s) in (\"\")"=w241) -> ("States Out"=w240:string)  [unwired: 13 in]
          }
          frame "---------- Process ----------" {
            # "Template Separator\n(You can make a copy of, or modify, this frame)"
            n80 = call <vilib>:"Add State(s) to Queue__jki_lib_state_machine.vi"("State(s) in (\"\")"=w246) -> ("States Out"=w245:string)  [unwired: 14 in]
          }
          frame "Process: Sync" {
            n81 = Unbundle By Name(w254) -> ("Self Reference"=w250:refnum<class "Chart[Template].lvclass">)
            n82 = call <vilib>:"WaitOnProcessSync.vi"("error in (no error)"=w249, "SMO"=w250) -> ("error out"=w248:errorcluster, "Don't run?"=w253:bool)  [unwired: 7 in, 1 out]
            n83 = Select(t="Data: Cleanup\nEvents: Unregister\nExit", s=w253, f="") -> (s? t:f=w247:string)
            n84 = call <vilib>:"Add State(s) to Queue__jki_lib_state_machine.vi"("State(s) in Front (\"\")"=w247, "State(s) in (\"\")"=w257) -> ("States Out"=w256:string)  [unwired: 13 in]
          }
          frame "---------- Events ----------" {
            # "Template Separator\n(You can make a copy of, or modify, this frame)"
            n85 = call <vilib>:"Add State(s) to Queue__jki_lib_state_machine.vi"("State(s) in (\"\")"=w262) -> ("States Out"=w261:string)  [unwired: 14 in]
          }
          frame "Events: Register" {
            w266 = cluster{"New Value":refnum<user-event>} {"New Value"=refnum}  # Dependency.PublicEvents
            # "Get Event from SMO"
            # "Register for Data Producer Event here..."
            n86 = Unbundle By Name(w279) -> ("Self Reference"=w272:refnum<class "Chart[Template].lvclass">)
            n87 = call <vilib>:"GetProtectedEvents.vi"("SMO"=w272) -> ("error out"=w264:errorcluster, "SMO Protected Events"=w277:T6)  [unwired: 8 in, 1 out]
            n88 = call "Chart[Template].GetProtectedEvents.vi"("Chart[Template]"=w272) -> ("error out"=w265:errorcluster, "Protected Events"=w274:T7)  [unwired: 8 in, 1 out]
            n89 = call "Chart[Template].GetDependencies.vi"("Chart[Template]"=w272) -> ("error out"=w263:errorcluster, "Dependencies"=w270:T8)  [unwired: 8 in, 1 out]
            n90 = Unbundle By Name(w270) -> ("SMO"=w268:refnum<class "SMO.lvclass">, "New Value"=w267:refnum<user-event>)
            n91 = Not A Number/Path/Refnum?(number/path/refnum=w267) -> (NaN/Path/Refnum?=w269:bool)
            n92 = case shown="True" w269 {
              tunnel: w268 -> [_ _]
              tunnel: w267 -> [w282 _]
              tunnel: w266 -> [w284 w287]
              tunnel: [w283 w286] -> w273
              frame False {
                n93 = Bundle By Name(cluster=w284, "New Value"=w282) -> (w283:cluster{"New Value":refnum<user-event>})
              }
              frame True {
                n94 = Bundle By Name(cluster=w287, "New Value"=refnum<user-event> refnum) -> (w286:cluster{"New Value":refnum<user-event>})
              }
            }
            n95 = register-events(w277, w274, w273) -> (reference out=w278:refnum<event-registration>, error out=w275:errorcluster)  [unwired: 2 in]
            n96 = Merge Errors(w271, w275, w263, w264, w265) -> (w276:errorcluster)
            n97 = call <vilib>:"Add State(s) to Queue__jki_lib_state_machine.vi"("State(s) in (\"\")"=w281) -> ("States Out"=w280:string)  [unwired: 14 in]
          }
          frame "Events: Unregister" {
            n98 = Unregister For Events(event registration refnum=w290, error in=w289) -> (error out=w288:errorcluster)
            n99 = call <vilib>:"Clear Errors.vi"("error in (no error)"=w288) -> ()  [unwired: 6 in, 1 out]
            n100 = call <vilib>:"Add State(s) to Queue__jki_lib_state_machine.vi"("State(s) in (\"\")"=w293) -> ("States Out"=w292:string)  [unwired: 14 in]
          }
          frame "---------- Action ----------" {
            n101 = call <vilib>:"Add State(s) to Queue__jki_lib_state_machine.vi"("State(s) in (\"\")"=w298) -> ("States Out"=w297:string)  [unwired: 14 in]
          }
          frame "Action: Clear Chart" {
            n102 = Unbundle By Name(w302) -> ("Self Reference"=w299:refnum<class "Chart[Template].lvclass">)
            n103 = call-dynamic "Chart[Template].Clear.vi"("error in (no error)"=w301, "Chart[Template]"=w299) -> ("error out"=w300:errorcluster)  [unwired: 8 in, 1 out]
            n104 = call <vilib>:"Add State(s) to Queue__jki_lib_state_machine.vi"("State(s) in (\"\")"=w305) -> ("States Out"=w304:string)  [unwired: 14 in]
          }
          frame "Action: Notify UI Closed" {
            # "Notify that the UI has been closed"
            n105 = Unbundle By Name(w308) -> ("Self Reference"=w309:refnum<class "Chart[Template].lvclass">)
            n106 = call <vilib>:"Hide.vi"("error in (no error)"=w307, "SMO.UI"=w309) -> ("error out"=w306:errorcluster)  [unwired: 8 in, 1 out]
            n107 = call <vilib>:"Add State(s) to Queue__jki_lib_state_machine.vi"("State(s) in (\"\")"=w312) -> ("States Out"=w311:string)  [unwired: 14 in]
          }
        }
      }
    }
    frame Error {
    }
  }
  n108 = call-parent "Process.vi"("error in (no error)"=w8, "SMO.UI"=w7) -> ("error out"=w5:errorcluster, "SMO.UI out"=→"Graph[Template] out":refnum<class "Chart[Template].lvclass">)  [unwired: 8 in]
  n109 = Merge Errors(w5, w4) -> (→"error out":errorcluster)
